vi "week04_Ex03.vi"() -> ()   [LabVIEW 2017]
panel:
  out "length":i32
  in  "String":string
  out "All i condition":i32[](array[numeric])
  out "Last i":i32
  out "All i comdition":i32[](array[numeric])
  out "LAST i":i32
  out "i":i32
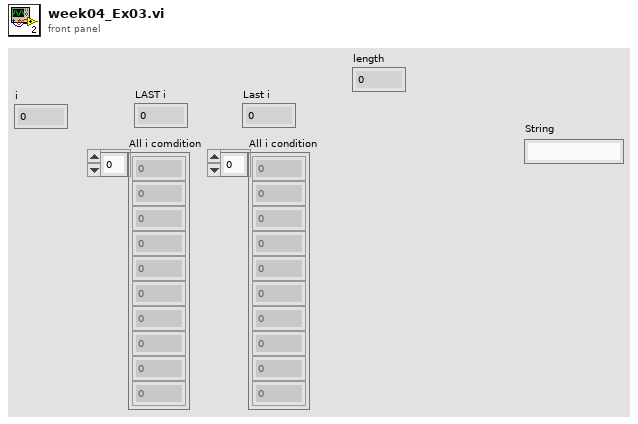
[diagram p1: front panel]
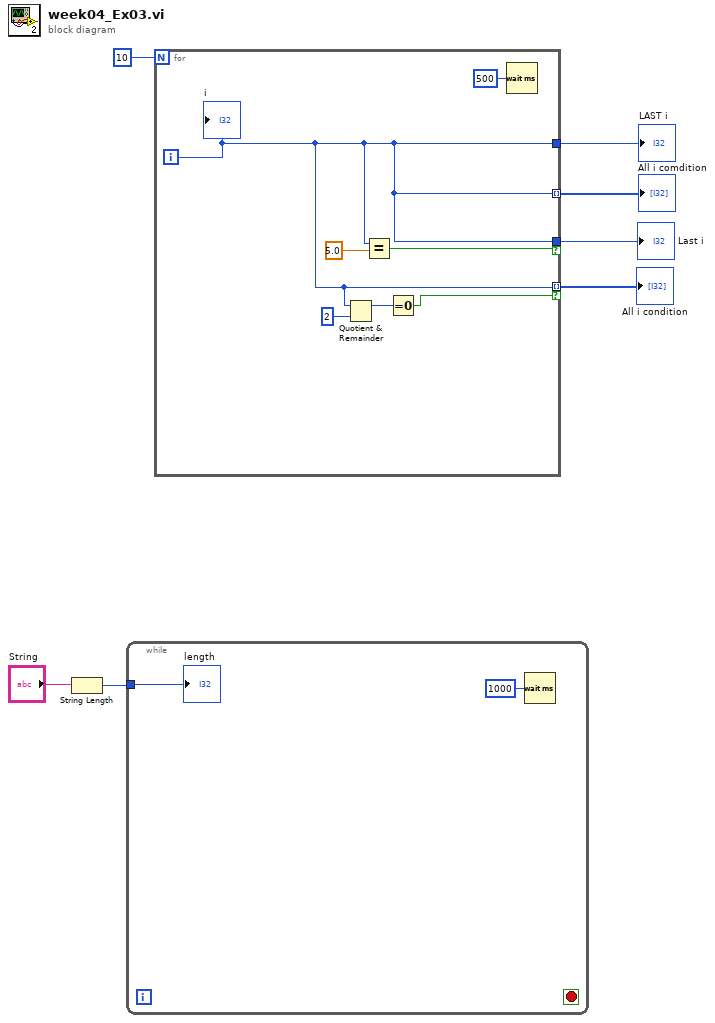
[diagram p0: block diagram]
diagram:
  n1 = String Length(string="String") -> (length=w1:i32)
  n2 = while {
    tunnel: w1 -> [w8]
    stop <- _ stop-if-true
    n3 = Wait (ms)(milliseconds to wait=u32 1000) -> ()  [unwired: 1 out]
    "length" <- w8
  }
  n4 = for {
    N: 10 -> [_]
    tunnel: [w13] -> w6
    tunnel: [w13] -> w5 mode=indexing
    tunnel: [w13] -> w4 if=w15
    tunnel: [w13] -> w3 mode=indexing if=w10
    i -> [w13]
    n5 = Quotient & Remainder(x=w13, y=2) -> (x-y*floor(x/y)=w11:i32)  [unwired: 1 out]
    n6 = Equal?(x=w13, y=5.0) -> (x = y?=w15:bool)
    n7 = Equal To 0?(x=w11) -> (x = 0?=w10:bool)
    n8 = Wait (ms)(milliseconds to wait=u32 500) -> ()  [unwired: 1 out]
    "i" <- w13
  }
  "LAST i" <- w6
  "All i comdition" <- w5
  "Last i" <- w4
  "All i condition" <- w3
